vi "TimeInterpBoolean_PopOldestSample.vi"(11 "in TimeInterpBoolean":T1) -> (0 "Is Present":bool, 1 "TimeStamp":dbl, 2 "OutputBoolean":bool, 3 "out TimeInterpBoolean":T1)   [LabVIEW 2019, in "Trajectory_Library.lvlib"]
doc: "Sample the buffer at the given time.\n\nInputs:\n - TimeInterpVariant -- Input data cluster\n - TimeStamp -- Time at which to sample (seconds)\n\nOutputs\n - OutputPose -- Sampled Variant. This is an exact value if there is a sample in the buffer at this time. Otherwise the value is interpolated. A custom routine will need to be called to extract the custom data from the variant. \n - IsPresent -- Returns TRUE if the buffer contains data as far back as TimeStamp."
uses:
  Trajectory_Library.lvlib
  TypeDef/TIME_INTERPOLATABLE_BOOLEAN.ctl
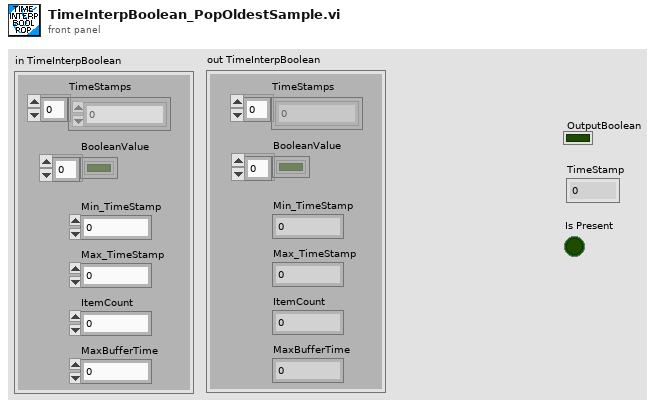
[diagram p1: front panel]
types:
  T1 = typedef "Trajectory_Library.lvlib/TIME_INTERPOLATABLE_BOOLEAN.ctl" = cluster{"TimeStamps":dbl[], "BooleanValue":bool[], "Min_TimeStamp":dbl, "Max_TimeStamp":dbl, "ItemCount":i32, "MaxBufferTime":dbl}
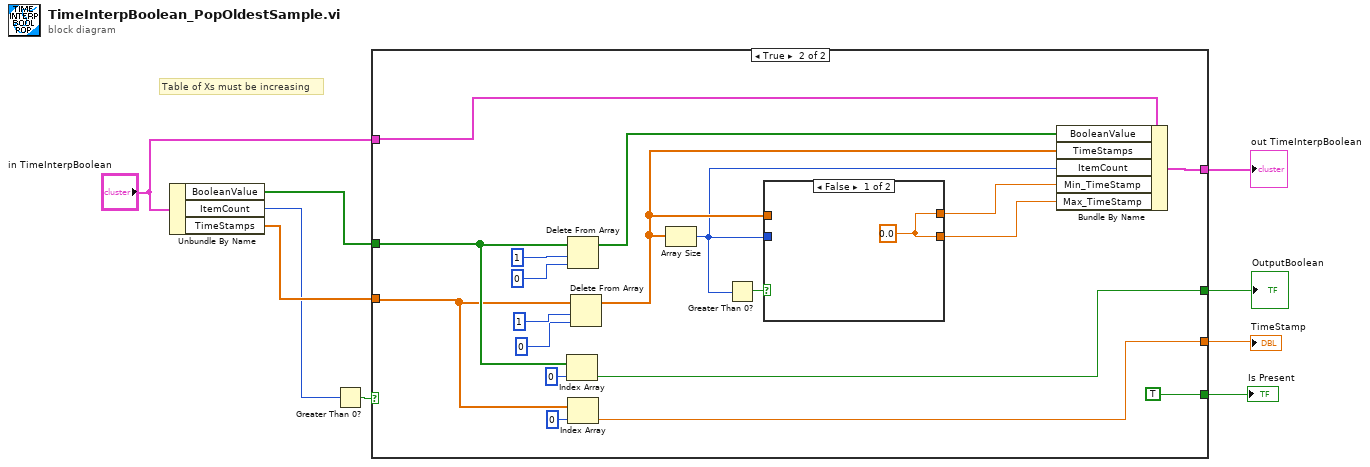
[diagram p0: block diagram]
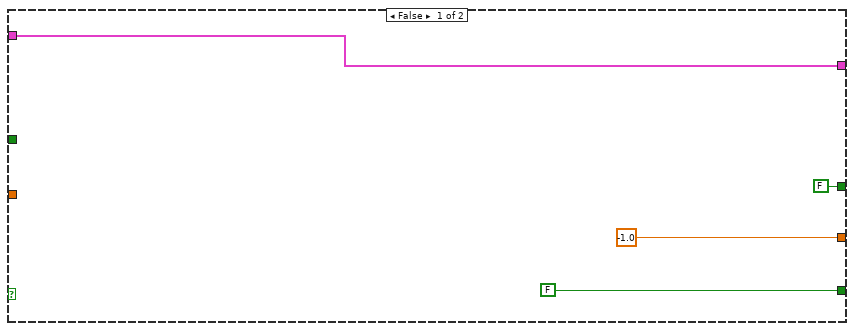
[diagram p2: hidden frame]
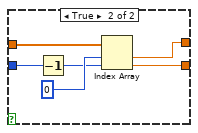
[diagram p3: hidden frame]
diagram:
  # "Table of Xs must be increasing"
  n1 = Unbundle By Name("in TimeInterpBoolean") -> ("BooleanValue"=w8:bool[], "ItemCount"=w6:i32, "TimeStamps"=w9:dbl[])
  n2 = Greater Than 0?(x=w6) -> (x > 0?=w7:bool)
  n3 = case shown="True" w7 {
    tunnel: [FALSE ("Table Y") w21] -> w5
    tunnel: w9 -> [_ w23]
    tunnel: w8 -> [_ w25]
    tunnel: [w13 w27] -> w4
    tunnel: "in TimeInterpBoolean" -> [w13 w28]
    tunnel: [FALSE TRUE] -> w2
    tunnel: [-1.0 w18] -> w1
    frame False {
    }
    frame True {
      n4 = Index Array(array=w25, index=0) -> (element=w21:bool)
      n5 = Delete From Array(array=w25, length=1, index=0) -> (array with subset deleted=w26:bool[])  [unwired: 1 out]
      n6 = Index Array(array=w23, index=0) -> (element=w18:dbl)
      n7 = Delete From Array(array=w23, length=1, index=0) -> (array with subset deleted=w20:dbl[])  [unwired: 1 out]
      n8 = Array Size(array=w20) -> (size(s)=w16:i32)
      n9 = Greater Than 0?(x=w16) -> (x > 0?=w17:bool)
      n10 = case shown="False" w17 {
        tunnel: w20 -> [_ w38]
        tunnel: w16 -> [_ w36]
        tunnel: [w33 w35] -> w15
        tunnel: [w33 w34] -> w14
        frame False {
          w33 = 0.0 ("Table X")
        }
        frame True {
          n11 = Decrement(x=w36) -> (x-1=w37:i32)
          n12 = Index Array(array=w38, index #1=0 ("index"), index #2=w37) -> (element #1=w35:dbl, element #2=w34:dbl)
        }
      }
      n13 = Bundle By Name(cluster=w28, "BooleanValue"=w26, "TimeStamps"=w20, "ItemCount"=w16, "Min_TimeStamp"=w15, "Max_TimeStamp"=w14) -> (w27:T1)
    }
  }
  "OutputBoolean" <- w5
  "out TimeInterpBoolean" <- w4
  "Is Present" <- w2
  "TimeStamp" <- w1
